vi "Apparent Power.vi"(4 "Arms":dbl=0.001 format="%#_13g", 5 "Vrms":dbl=0.001 format="%#_13g") -> (1 "Apparent Power":dbl)   [LabVIEW 2014]
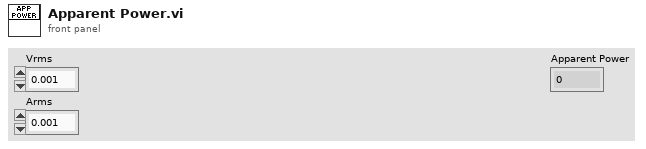
[diagram p1: front panel]
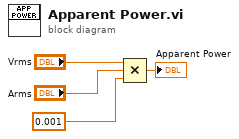
[diagram p0: block diagram]
diagram:
  n1 = Compound Arithmetic op=MULTIPLY("Vrms", "Arms", 0.001 ("Vrms 2")) -> (→"Apparent Power":dbl)
